vi "Priority.vi"(8 "error in (no error)":errorcluster, 11 "SSE Handler in":refnum<class "SSE Handler.lvclass">) -> (0 "error out":errorcluster, 2 "Priority":u16, 3 "SSE Handler out":refnum<class "SSE Handler.lvclass">)   [LabVIEW 2020, in "HTTP Server.lvlib" / "SSE Handler.lvclass"]
doc: "Determines the order that handlers are run during each processing step. Handlers are sorted numerically so that lower number priorities will run before higher numbered priorities. The default priority is 10000 with a maximum value of 65535. Most built-in authentication priorities are below 200, websocket request checks happen at 1000, fallback handlers such as file and cache serving are at 30000, and most built-in response finalization runs at 60000+"
uses:
  SSE Handler.lvclass
  SSE Handler.lvclass/SSE Handler.ctl
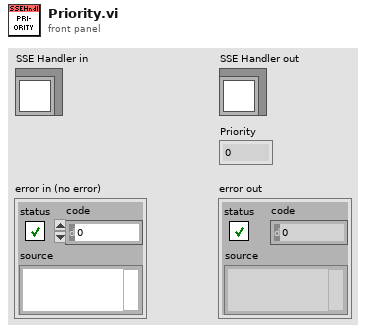
[diagram p1: front panel]
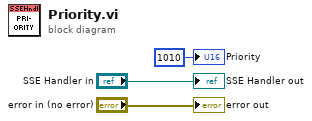
[diagram p0: block diagram]
diagram:
  "error out" <- "error in (no error)"
  "SSE Handler out" <- "SSE Handler in"
  "Priority" <- u16 1010 ("Priority")
